vi "Read.vi"(0 "Smart_Eye_Pro_Driver in":refnum<class "SmartEyeProDriver.lvclass">, 5 "max size (548)":i32=548, 11 "error in (no error)":errorcluster) -> (3 "Sync Id":u32, 4 "Smart_Eye_Pro_Driver out":refnum<class "SmartEyeProDriver.lvclass">, 6 "Data out":refnum<class "Data.lvclass">, 8 "Packet type":u16, 10 "Packet length":u16, 15 "error out":errorcluster)   [LabVIEW 2020, in "SmartEyeProDriver.lvclass"]
uses:
  SmartEyeProDriver.lvclass
  Data Class/Data.lvclass
  SmartEyeProDriver.lvclass/SmartEyeProDriver.ctl
  Decode Class/FrameInfo_class/FrameInfo.lvclass
  C:/Users/theod/Desktop/API - EyeT data streaming to IC/Smart Eye API/Source/Classes/Smart Eye Pro Drivers/Decode Class/Decode_Packet/Decode_Packet.lvclass
  Decode Class/Gaze_class/Gaze.lvclass
  Decode Class/Pupil_class/Pupil.lvclass
  Decode Class/AllInOne_class/AllInOne.lvclass
  Decode Class/Decode_Packet/Decode_Packet.lvclass
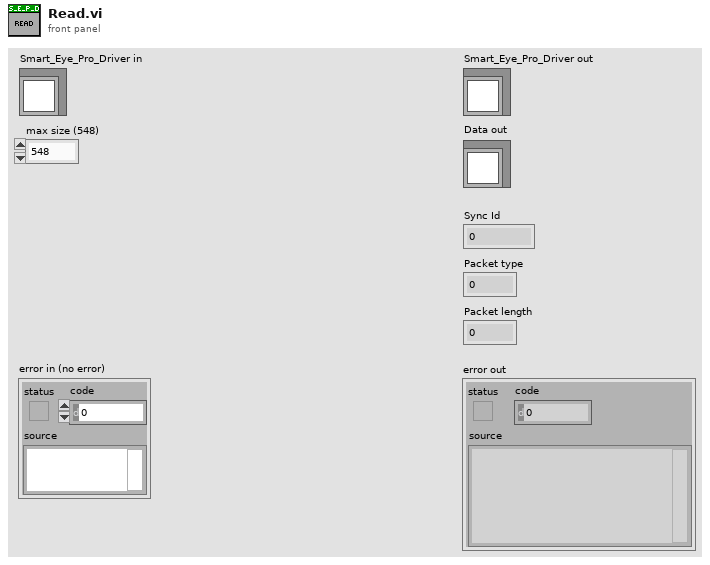
[diagram p1: front panel]
types:
  T1 = typedef "Decode_Packet.lvclass/Decode_type.ctl" = enum16{"Frame Information", "Raw Gaze", "Pupilometry", "All In One"}
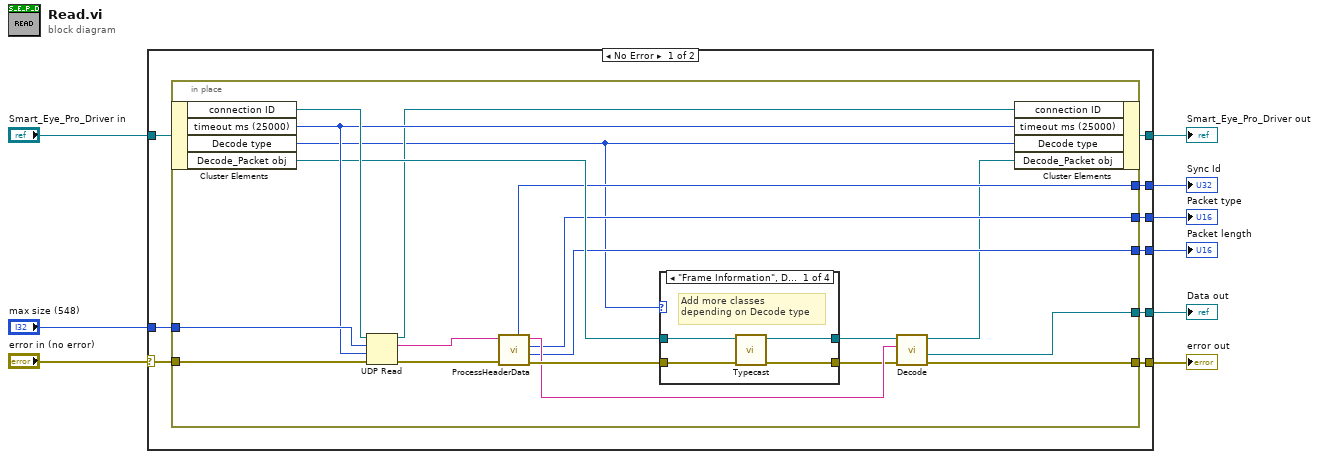
[diagram p0: block diagram]
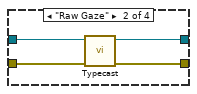
[diagram p2: hidden frame]
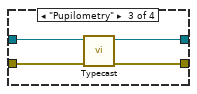
[diagram p3: hidden frame]
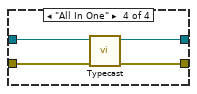
[diagram p4: hidden frame]
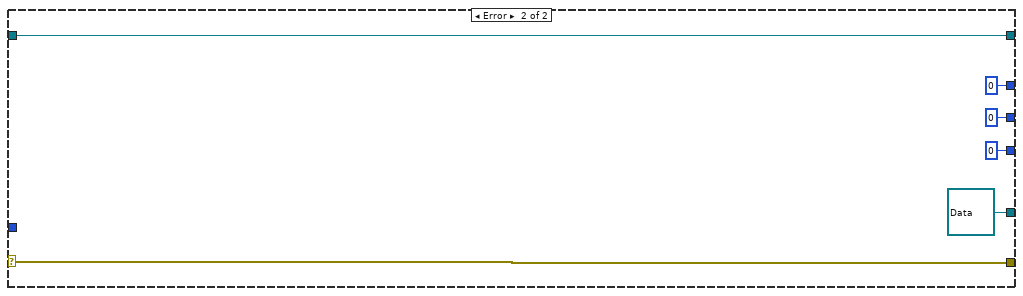
[diagram p5: hidden frame]
diagram:
  n1 = case shown="No Error" "error in (no error)" {
    selector: "error in (no error)" -> [w17 w59]
    tunnel: [w15 w59] -> w8
    tunnel: [w14 w58] -> w6
    tunnel: "Smart_Eye_Pro_Driver in" -> [w18 w58]
    tunnel: "max size (548)" -> [w16 _]
    tunnel: [w13 u16 0 ("Packet length")] -> w4
    tunnel: [w12 u16 0 ("Packet type")] -> w3
    tunnel: [w11 u32 0 ("Sync Id")] -> w2
    tunnel: [w10 refnum<class "Data.lvclass"> refnum] -> w1
    frame No Error {
      n2 = in-place {
        in-place-border: w17 -> [w36]
        in-place-border: w16 -> [w35]
        in-place-border: [w33] -> w15
        in-place-border: [w32] -> w10
        in-place-border: [w25] -> w13
        in-place-border: [w24] -> w12
        in-place-border: [w23] -> w11
        n3 = in-place-cluster #1(w18) -> ("connection ID"=w37:refnum<k16>, "timeout ms (25000)"=w34:i32, "Decode type"=w19:T1, "Decode_Packet obj"=w27:refnum<class "Decode_Packet.lvclass">)
        n4 = UDP Read(connection ID=w37, max size (548)=w35, timeout ms (25000)=w34, 8:w36) -> (data out=w29:string, error out=w31:errorcluster, 3:w26:refnum<k16>)  [unwired: 2 out]
        n5 = call "ProcessHeaderData.vi"("error in"=w31, "Binary string"=w29) -> ("error out"=w30:errorcluster, "Packet length"=w25:u16, "Packet type"=w24:u16, "Binary string without header"=w28:string, "Sync Id"=w23:u32)  [unwired: 5 in]
        n6 = case shown="\"Frame Information\", Default" w19 {
          tunnel: w30 -> [w39 w43 w47 w52]
          tunnel: [w38 w42 w46 w51] -> w20
          tunnel: [w40 w44 w48 w50] -> w21
          tunnel: w27 -> [w41 w45 w49 w53]
          frame "Frame Information", Default {
            # "Add more classes\ndepending on Decode type"
            n7 = call "Typecast.vi"("error in (no error)"=w39, "Decode_Packet in"=w41) -> ("error out"=w38:errorcluster, "General out"=w40:refnum<class "FrameInfo.lvclass">)  [unwired: 8 in]
          }
          frame "Raw Gaze" {
            n8 = call "Typecast.vi"("error in (no error)"=w43, "Decode_Packet in"=w45) -> ("error out"=w42:errorcluster, "Pupil_Diameter out"=w44:refnum<class "Gaze.lvclass">)  [unwired: 8 in]
          }
          frame "Pupilometry" {
            n9 = call "Typecast.vi"("error in (no error)"=w47, "Decode_Packet in"=w49) -> ("error out"=w46:errorcluster, "Pupil_Diameter out"=w48:refnum<class "Pupil.lvclass">)  [unwired: 8 in]
          }
          frame "All In One" {
            n10 = call "Typecast.vi"("error in (no error)"=w52, "Decode_Packet in"=w53) -> ("error out"=w51:errorcluster, "Pupil_Diameter out"=w50:refnum<class "AllInOne.lvclass">)  [unwired: 8 in]
          }
        }
        n11 = call-dynamic "Decode.vi"("error in (no error)"=w20, "Binary string in"=w28, "obj in"=w21) -> ("error out"=w33:errorcluster, "Data out"=w32:refnum<class "Data.lvclass">, "obj out"=w22:refnum<class "Decode_Packet.lvclass">)  [unwired: 5 in, 1 out]
        n12 = in-place-cluster #1("connection ID"=w26, "timeout ms (25000)"=w34, "Decode type"=w19, "Decode_Packet obj"=w22) -> (w14:refnum<class "SmartEyeProDriver.lvclass">)
      }
    }
    frame Error {
    }
  }
  "error out" <- w8
  "Smart_Eye_Pro_Driver out" <- w6
  "Packet length" <- w4
  "Packet type" <- w3
  "Sync Id" <- w2
  "Data out" <- w1
